vi "Experiment 9.vi"() -> ()   [LabVIEW 2026]
doc: "Experiment 9"
uses:
  <vilib>/Analysis/NI_AALBase.lvlib
  <vilib>/Analysis/baseanly.llb/Mean (DBL).vi
panel:
  out "Avg. No. Of Iterations Executed - All Loops":dbl format="%.1f"
  out "No. Of Iterations Executed - Loop 2":i32
  out "Output - Loop 2":dbl[](array[numeric]) format="%.3f"
  out "No. Of Iterations Executed - Loop 1":i32
  out "Output - Loop 1":dbl[](array[numeric]) format="%.3f"
  out "Stop VI?":bool
  # "Experiment 9"
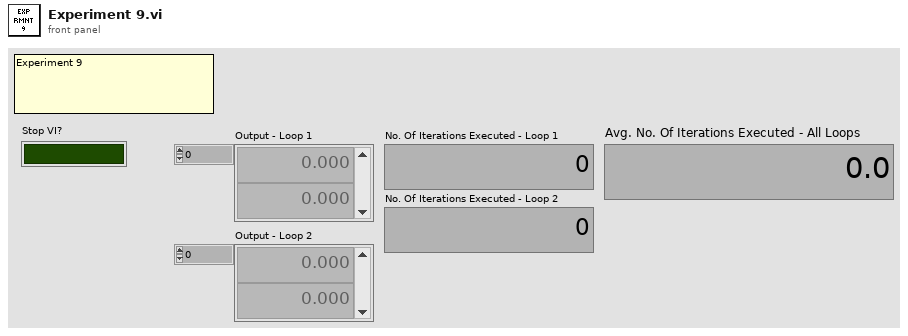
[diagram p1: front panel]
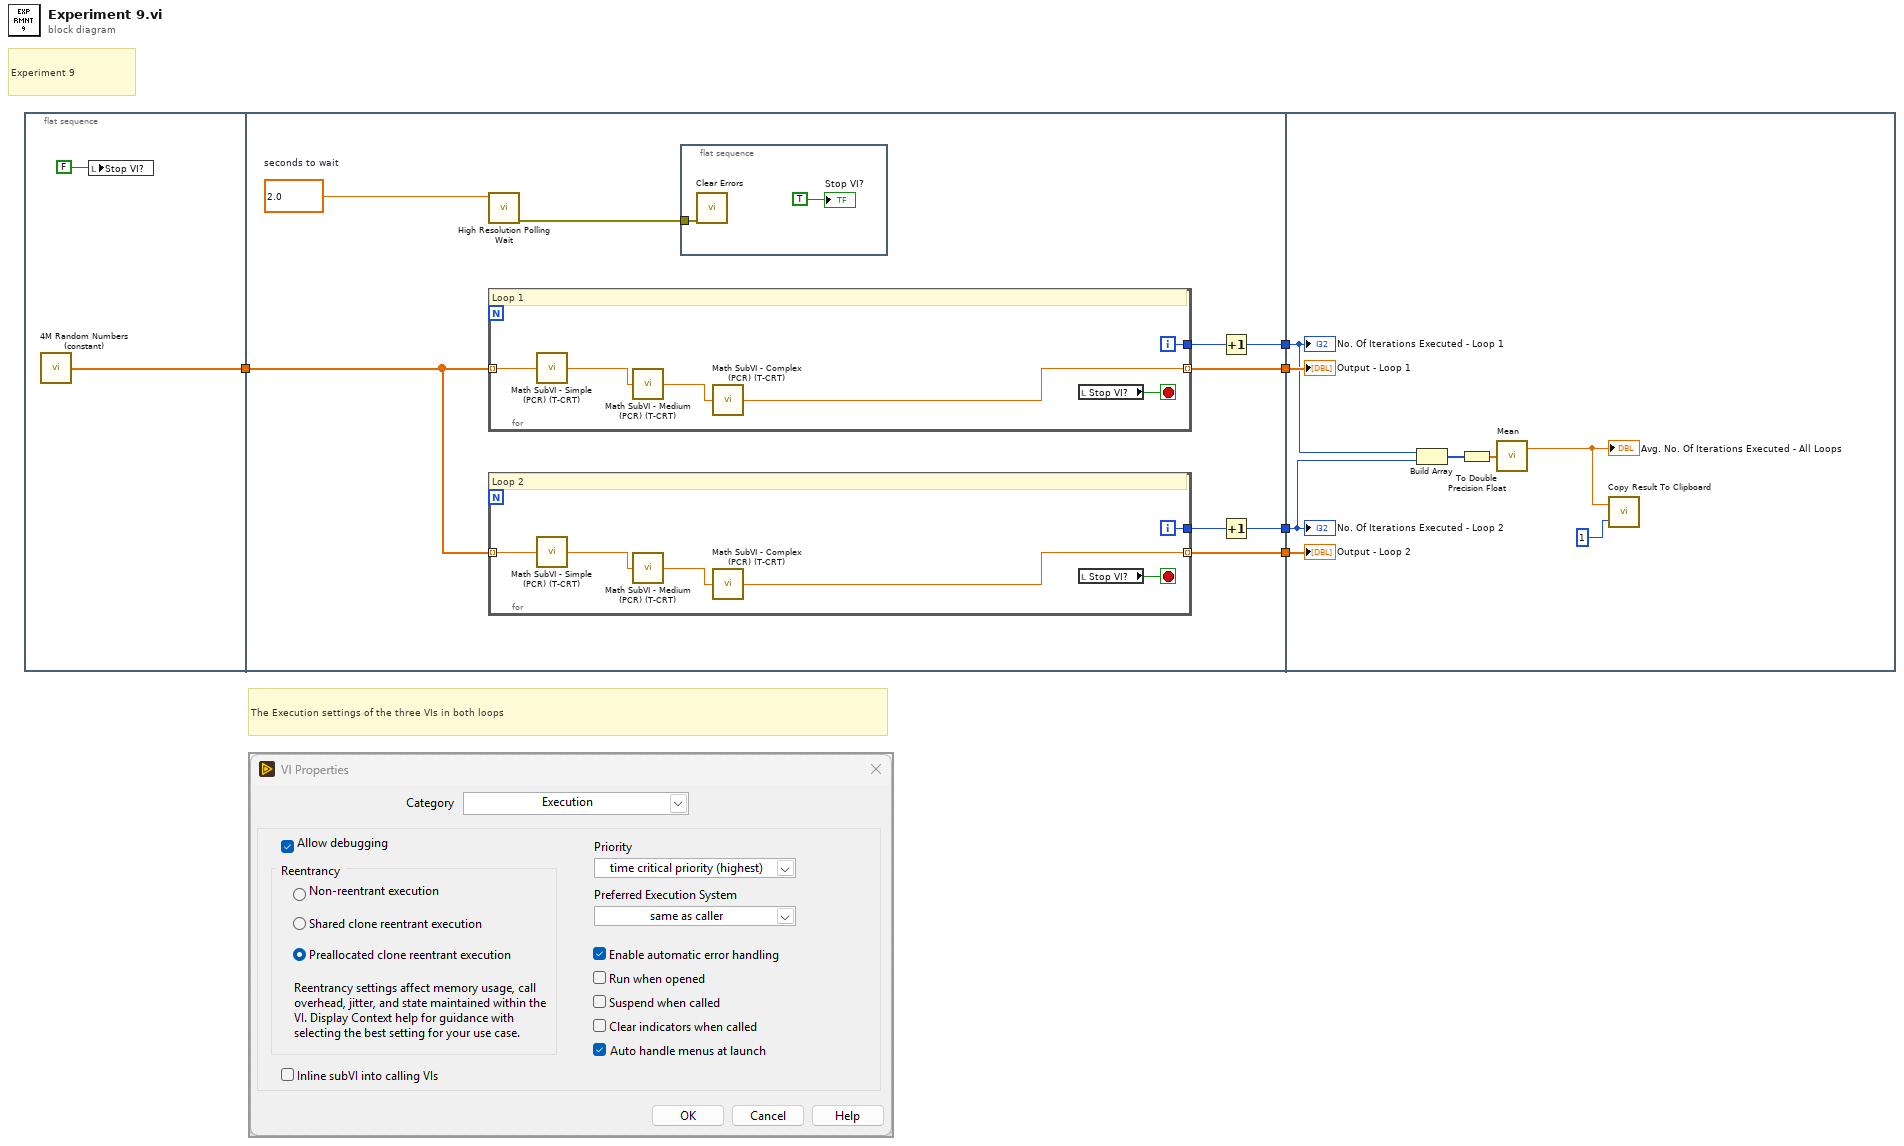
[diagram p0: block diagram]
diagram:
  # "The Execution settings of the three VIs in both loops"
  # "Experiment 9"
  n1 = flat-sequence {
    tunnel: [w6] -> w1
    tunnel: [w9] -> w5
    tunnel: [w14] -> w4
    tunnel: [w13] -> w3
    tunnel: [w11] -> w2
    tunnel: w1 -> [w10]
    tunnel: w5 -> [w38]
    tunnel: w4 -> [w32]
    tunnel: w3 -> [w31]
    tunnel: w2 -> [w37]
    frame #0 {
      n2 = call "4M Random Numbers (constant).vi"() -> ("4M Random Numbers"=w6:dbl[])
      n3 = local write "Stop VI?"(FALSE) -> ()
    }
    frame #1 {
      w16 = 2.0  # seconds to wait
      n4 = call <vilib>:"High Resolution Polling Wait.vi"("seconds to wait"=w16) -> ("error out"=w15:errorcluster)  [unwired: 10 in]
      n5 = for {
        tunnel: w10 -> [w20] mode=indexing
        tunnel: [w19] -> w9 mode=indexing
        tunnel: [w21] -> w8
        i -> [w21]
        stop <- w22 stop-if-true
        # "Loop 1"
        n6 = call "Math SubVI - Simple (PCR) (T-CRT).vi"("Input"=w20) -> ("Output"=w17:dbl)
        n7 = call "Math SubVI - Medium (PCR) (T-CRT).vi"("Input"=w17) -> ("Output"=w18:dbl)
        n8 = call "Math SubVI - Complex (PCR) (T-CRT).vi"("Input"=w18) -> ("Output"=w19:dbl)
        n9 = local read "Stop VI?"() -> (w22:bool)
      }
      n10 = for {
        tunnel: w10 -> [w26] mode=indexing
        tunnel: [w25] -> w11 mode=indexing
        tunnel: [w27] -> w12
        i -> [w27]
        stop <- w28 stop-if-true
        # "Loop 2"
        n11 = call "Math SubVI - Simple (PCR) (T-CRT).vi"("Input"=w26) -> ("Output"=w23:dbl)
        n12 = call "Math SubVI - Medium (PCR) (T-CRT).vi"("Input"=w23) -> ("Output"=w24:dbl)
        n13 = call "Math SubVI - Complex (PCR) (T-CRT).vi"("Input"=w24) -> ("Output"=w25:dbl)
        n14 = local read "Stop VI?"() -> (w28:bool)
      }
      n15 = flat-sequence {
        tunnel: w15 -> [w29]
        frame #0 {
          n16 = call <vilib>:"Clear Errors.vi"("error in (no error)"=w29) -> ()  [unwired: 5 in, 2 out]
          "Stop VI?" <- TRUE
        }
      }
      n17 = Increment(x=w8) -> (x+1=w14:i32)
      n18 = Increment(x=w12) -> (x+1=w13:i32)
    }
    frame #2 {
      n19 = Build Array(w32, w31) -> (w34:i32[])
      n20 = To Double Precision Float(number=w34) -> (double precision float=w33:dbl[])
      n21 = call-poly <vilib>:"Mean.vi"("X"=w33) -> ("mean"=w36:dbl)  [unwired: 1 out]
      "Avg. No. Of Iterations Executed - All Loops" <- w36
      n22 = call "Copy Result To Clipboard.vi"("No. Of Decimal Places (6)"=u32 1, "Input"=w36) -> ()
      "No. Of Iterations Executed - Loop 1" <- w32
      "Output - Loop 1" <- w38
      "No. Of Iterations Executed - Loop 2" <- w31
      "Output - Loop 2" <- w37
    }
  }
